vi "Analysator Definition 2 String Array.vi"(11 "AnalysatorDefinition Array in":T1[](array[typedef])) -> (3 "Analysator String Array":string[][](array[string]))   [LabVIEW 2020, in "System Einstellungen V2.lvlib"]
uses:
  System Einstellungen V2.lvlib
  AnalysatorDefinition.ctl
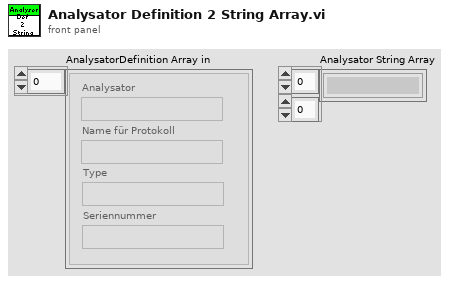
[diagram p1: front panel]
types:
  T1 = typedef "System Einstellungen V2.lvlib/AnalysatorDefinition.ctl" = cluster{"Analysator":string, "Name für Protokoll":string, "Type":string, "Seriennummer":string}
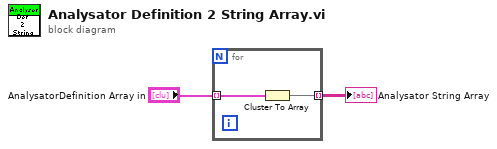
[diagram p0: block diagram]
diagram:
  n1 = for {
    tunnel: "AnalysatorDefinition Array in" -> [w4] mode=indexing
    tunnel: [w3] -> w1 mode=indexing
    n2 = Cluster To Array(cluster=w4) -> (array=w3:string[])
  }
  "Analysator String Array" <- w1
